vi "DbdPathName.vi"() -> (0 "pathName":string)   [LabVIEW 2018]
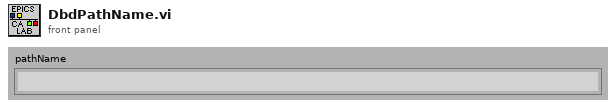
[diagram p1: front panel]
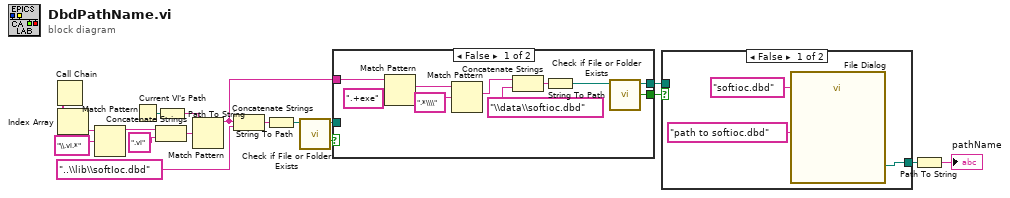
[diagram p0: block diagram]
diagram:
  n1 = Call Chain() -> (call chain=w17:string[])
  n2 = Index Array(array=w17) -> (element=w15:string)  [unwired: 1 in]
  n3 = Match Pattern(string=w15, regular expression="\\.vi.*") -> (before substring=w14:string)  [unwired: 4 out]
  n4 = Current VI's Path() -> (path=w18:path)
  n5 = Concatenate Strings(w14, ".vi" ("string")) -> (w12:string)
  n6 = Path To String(path=w18) -> (string=w11:string)
  n7 = Match Pattern(string=w11, regular expression=w12) -> (before substring=w6:string)  [unwired: 4 out]
  n8 = Concatenate Strings(w6, "..\\lib\\softIoc.dbd") -> (w9:string)
  n9 = String To Path(string=w9) -> (path=w10:path)
  n10 = call <vilib>:"Check if File or Folder Exists.vi"("path"=w10) -> ("file or folder exists?"=w8:bool, "dup path"=w7:path)  [unwired: 1 in, 8 out]
  n11 = case shown="False" w8 {
    selector: w8 -> [_ w29]
    tunnel: w7 -> [_ w30]
    tunnel: w6 -> [w20 _]
    tunnel: [w26 w30] -> w5
    tunnel: [w25 w29] -> w4
    frame False {
      n12 = Match Pattern(string=w20, regular expression=".+exe" ("search string")) -> (match substring=w22:string)  [unwired: 1 in, 3 out]
      n13 = Match Pattern(string=w22, regular expression=".*\\\\") -> (match substring=w19:string)  [unwired: 1 in, 3 out]
      n14 = Concatenate Strings(w19, "\\data\\softioc.dbd" ("string")) -> (w27:string)
      n15 = String To Path(string=w27) -> (path=w28:path)
      n16 = call <vilib>:"Check if File or Folder Exists.vi"("path"=w28) -> ("file or folder exists?"=w25:bool, "dup path"=w26:path)  [unwired: 1 in, 8 out]
    }
    frame True {
    }
  }
  n17 = case shown="False" w4 {
    tunnel: [w31 w34] -> w3
    tunnel: w5 -> [_ w34]
    frame False {
      n18 = call "File Dialog"("prompt"="path to softioc.dbd" ("pattern label"), "default name"="softioc.dbd") -> ("selected path"=w31:path)  [unwired: 5 in, 8 out]
    }
    frame True {
    }
  }
  n19 = Path To String(path=w3) -> (string=→"pathName":string)
